vi "GetFloatValue.vi"(2 "error in (no error)":errorcluster, 3 "Feature Name":string, 4 "IGxDevice":refnum<k24>) -> (0 "error out":errorcluster, 1 "Float Value":dbl)   [LabVIEW 2013, in "GxLVlib.lvlib"]
uses:
  GxLVlib.lvlib
  C:/Program Files/Daheng Imaging/GalaxySDK/Samples/LabVIEW SDK/x64/GxLVLib/dll/GxIAPINET.dll
  dll/GxIAPINET.dll
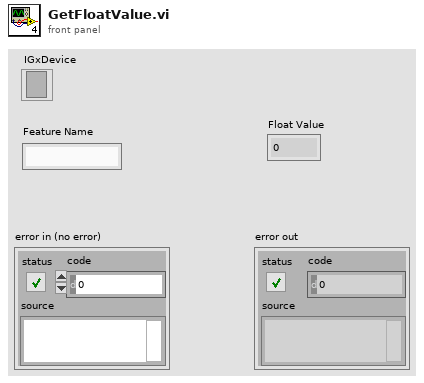
[diagram p1: front panel]
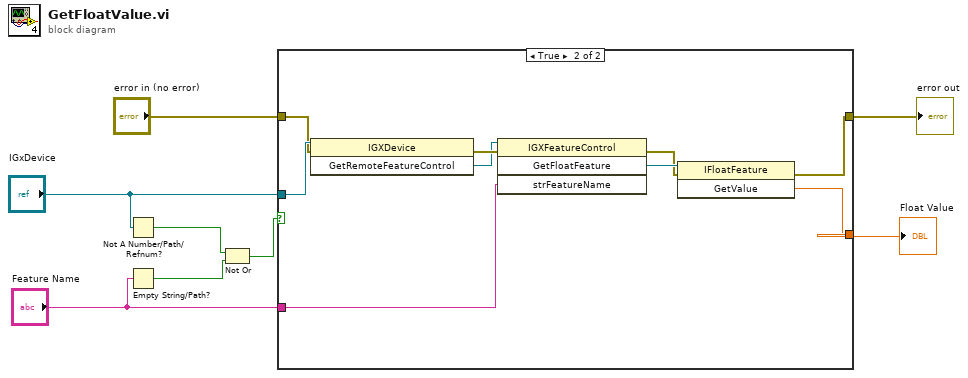
[diagram p0: block diagram]
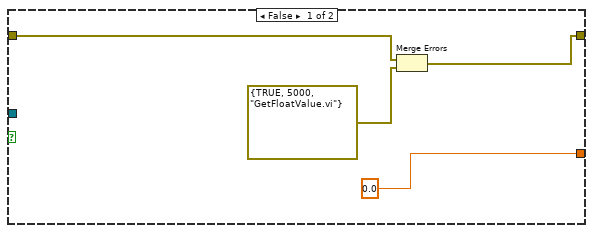
[diagram p2: hidden frame]
diagram:
  n1 = Not A Number/Path/Refnum?(number/path/refnum="IGxDevice") -> (NaN/Path/Refnum?=w8:bool)
  n2 = Empty String/Path?(string/path="Feature Name") -> (empty?=w7:bool)
  n3 = Not Or(1:w7, 2:w8) -> (0:w6:bool)
  n4 = case shown="True" w6 {
    tunnel: "error in (no error)" -> [w10 w20]
    tunnel: [w9 w13] -> w4
    tunnel: [0.0 w14] -> w3
    tunnel: "IGxDevice" -> [_ w21]
    tunnel: "Feature Name" -> [_ w18]
    frame False {
      n5 = Merge Errors(w10, errorcluster {TRUE, 5000, "GetFloatValue.vi"}) -> (w9:errorcluster)
    }
    frame True {
      n6 = invoke class="IGXDevice" method="GetRemoteFeatureControl"(reference=w21, error in=w20) -> (error out=w19:errorcluster, "GetRemoteFeatureControl"=w17:refnum<k24>)  [unwired: 1 in, 1 out]
      n7 = invoke class="IGXFeatureControl" method="GetFloatFeature"(reference=w17, error in=w19, "strFeatureName"=w18) -> (error out=w15:errorcluster, "GetFloatFeature"=w16:refnum<k24>)  [unwired: 1 in, 2 out]
      n8 = invoke class="IFloatFeature" method="GetValue"(reference=w16, error in=w15) -> (error out=w13:errorcluster, "GetValue"=w14:dbl)  [unwired: 1 in, 1 out]
    }
  }
  "error out" <- w4
  "Float Value" <- w3
